vi "Create Table.vi"(8 "error in (no error)":errorcluster) -> (0 "error out":errorcluster)   [LabVIEW 2020, in "Settings.lvlib"]
uses:
  Settings.lvlib
  <vilib>/drjdpowell/SQLite Library/SQL Connection/Open (path).vi
  <vilib>/drjdpowell/SQLite Library/SQL Connection/Open (string).vi
  <vilib>/AdvancedString/Path To Command Line String.vi
  <vilib>/drjdpowell/SQLite Library/SQL Connection/Execute SQL (No results).vi
  <vilib>/drjdpowell/SQLite Library/SQL Connection/Connection.lvclass
  <vilib>/drjdpowell/SQLite Library/SQLite.lvlib
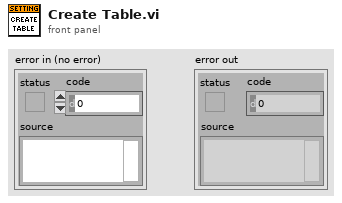
[diagram p1: front panel]
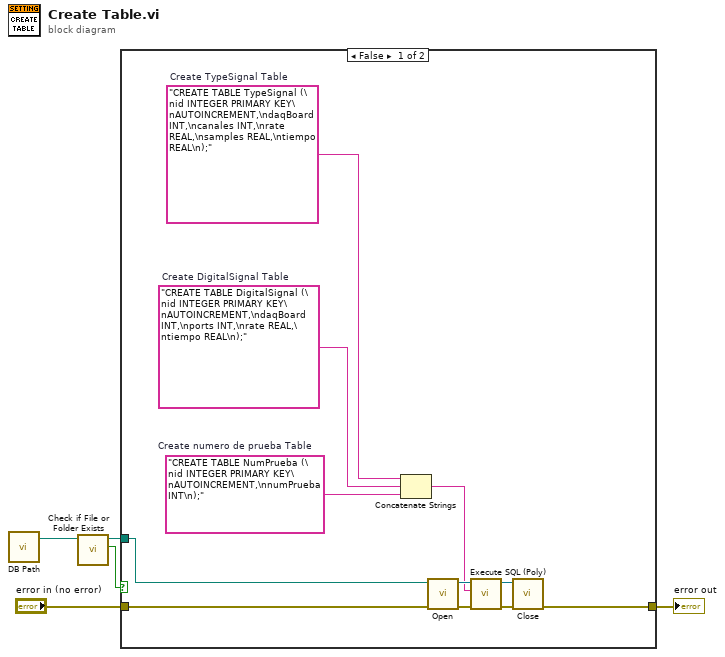
[diagram p0: block diagram]
diagram:
  n1 = call "DB Path.vi"() -> ("DB path"=w1:path)  [unwired: 11 in]
  n2 = call <vilib>:"Check if File or Folder Exists.vi"("path"=w1) -> ("file or folder exists?"=w5:bool, "dup path"=w4:path)  [unwired: 8 in, 1 out]
  n3 = case shown="False" w5 {
    tunnel: w4 -> [w12 _]
    tunnel: "error in (no error)" -> [w11 w17]
    tunnel: [w10 w17] -> w2
    frame False {
      w7 = "CREATE TABLE DigitalSignal (\nid INTEGER PRIMARY KEY\nAUTOINCREMENT,\ndaqBoard INT,\nports INT,\nrate REAL,\ntiempo REAL\n);"  # Create DigitalSignal Table
      w6 = "CREATE TABLE NumPrueba (\nid INTEGER PRIMARY KEY\nAUTOINCREMENT,\nnumPrueba INT\n);"  # Create numero de prueba Table
      w8 = "CREATE TABLE TypeSignal (\nid INTEGER PRIMARY KEY\nAUTOINCREMENT,\ndaqBoard INT,\ncanales INT,\nrate REAL,\nsamples REAL,\ntiempo REAL\n);"  # Create TypeSignal Table
      n4 = Concatenate Strings(w8, w7, w6) -> (w9:string)
      n5 = call-poly <vilib>:"Open.vi"("error in (no error)"=w11, "db file"=w12) -> ("error out"=w14:errorcluster, "SQLite Connection"=w15:refnum<class "Connection.lvclass">)  [unwired: 8 in]
      n6 = call-poly <vilib>:"Execute SQL (Poly).vi"("error in (no error)"=w14, "SQL"=w9, "SQLite Connection in"=w15) -> ("error out"=w13:errorcluster, "SQLite Connection"=w16:refnum<class "Connection.lvclass">)  [unwired: 7 in]
      n7 = call-dynamic "Close.vi"("error in (no error)"=w13, "SQLite Connection in"=w16) -> ("error out"=w10:errorcluster)  [unwired: 9 in]
    }
    frame True {
    }
  }
  "error out" <- w2
